vi "InitADCard.vi"(0 "task in":refnum<k21>, 1 "AD-Channels":string[](array[string]), 2 "reconfig (true)":bool=TRUE, 3 "Timing":T1={"AD-clock"=4000000.0, "external ADclock"=TRUE, "Galvocycle"=1e-05, "Bitsize"=1e-07, "AD.start.delay"=0.0, "AddStartTriggerIn"=FALSE, "VoltageRange"={"min Voltage"=-0.1, "max Voltage"=10.0}}, 4 "buffer size >1E6 (2.5E6)":i32=4000000, 5 "error in (no error)":errorcluster) -> (6 "task out":refnum<k21>, 7 "bit shifts up to 16bit":u8, 8 "error out":errorcluster)   [LabVIEW 2011]
uses:
  <vilib>/DAQmx/create/channels.llb/DAQmx Create Channel (AI-Voltage-Basic).vi
  <vilib>/DAQmx/configure/timing.llb/DAQmx Timing (Sample Clock).vi
  <vilib>/DAQmx/configure/trigger.llb/DAQmx Start Trigger (Digital Edge).vi
  National Instruments/LabVIEW 2011/resource/objmgr/daqmx.rc
panel:
  out "Trigger Pin":string
  out "8MHz Pin":string
  out "AI.RawSampJustification":i32(ring)=10279 items=["Right-Justified"=10279, "Left-Justified"=10209]
  out "RawDataWidth":u32
  out "NaN/Path/Refnum?":bool
  in  "trigger type (digital start)":enum16{"no trigger", "digital start"}(ring)=enum."digital start"
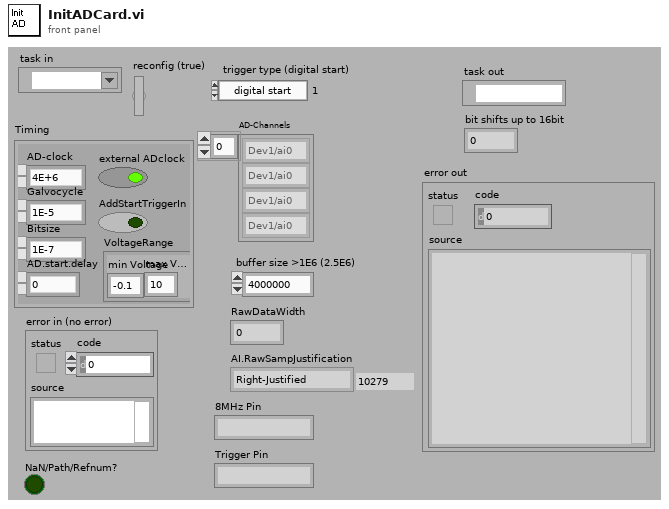
[diagram p1: front panel]
types:
  T1 = cluster{"AD-clock":dbl, "external ADclock":bool, "Galvocycle":dbl, "Bitsize":dbl, "AD.start.delay":dbl, "AddStartTriggerIn":bool, "VoltageRange":cluster{"min Voltage":dbl, "max Voltage":dbl}}
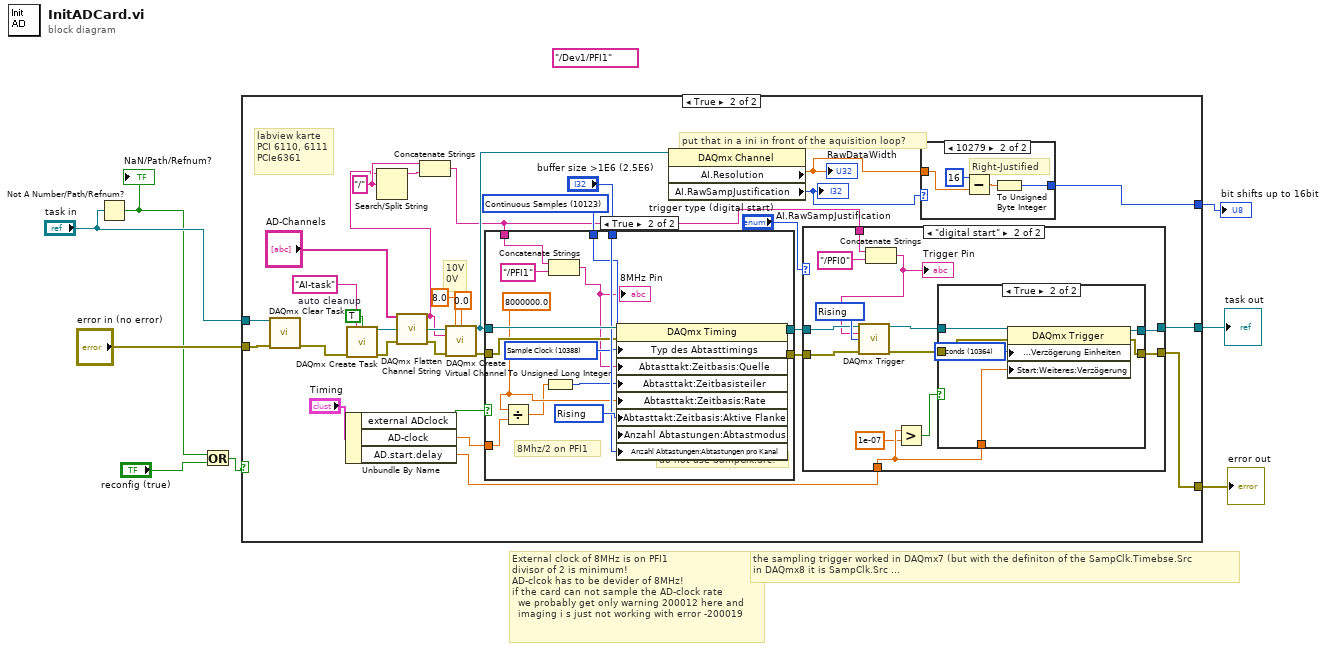
[diagram p0: block diagram]
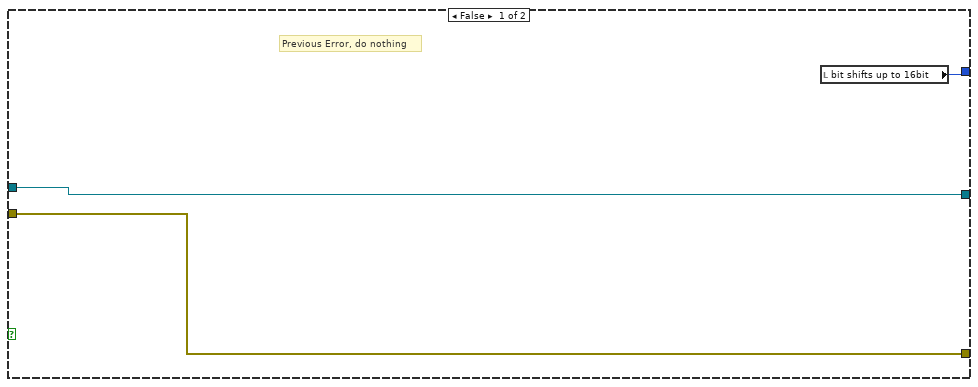
[diagram p2: hidden frame]
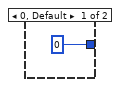
[diagram p3: hidden frame]
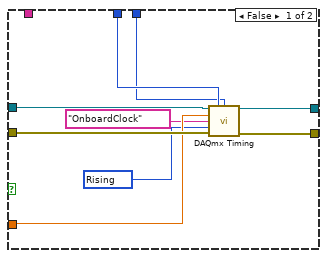
[diagram p6: hidden frame]
diagram:
  (unwired) tag "/Dev1/PFI1" ("source")
  # "External clock of 8MHz is on PFI1\ndivisor of 2 is minimum!\nAD-clcok has to be devider of 8MHz!\nif the card can not sample the AD-clock rate\n  we probably get only warning 200012 here and\n  imaging i s just not working with error -200019"
  # "the sampling trigger worked in DAQmx7 (but with the definiton of the SampClk.Timebse.Src\nin DAQmx8 it is SampClk.Src ..."
  n1 = Not A Number/Path/Refnum?(number/path/refnum="task in") -> (NaN/Path/Refnum?=w5:bool)
  "NaN/Path/Refnum?" <- w5
  n2 = Or(x=w5, y="reconfig (true)") -> (x .or. y?=w3:bool)
  n3 = case shown="True" w3 {
    tunnel: [w11 w29] -> w8
    tunnel: "error in (no error)" -> [w11 w21]
    tunnel: "task in" -> [w10 w20]
    tunnel: [w10 w23] -> w2
    tunnel: [w9 w16] -> w1
    frame False {
      # "Previous Error, do nothing"
      n4 = local read "bit shifts up to 16bit"() -> (w9:u8)
    }
    frame True {
      w14 = "/" ("search string/char (-)")
      w33 = 10123 items=["Finite Samples"=10178, "Continuous Samples"=10123, "Hardware Timed Single Point"=12522] ("sample mode")
      w41 = TRUE  # auto cleanup
      # "labview karte\nPCI 6110, 6111\nPCIe6361"
      # "put that in a ini in front of the aquisition loop?"
      # "10V\n0V"
      n5 = call <vilib>:"DAQmx Clear Task.vi"("task in"=w20, "error in"=w21) -> ("error out"=w22:errorcluster)  [unwired: 13 out]
      n6 = Unbundle By Name("Timing") -> ("external ADclock"=w26:bool, "AD-clock"=w25:dbl, "AD.start.delay"=w24:dbl)
      n7 = call <vilib>:"DAQmx Create Task.vi"("new task name"="AI-task", "auto cleanup"=w41, "error in"=w22) -> ("task out"=w40:refnum<k21>, "error out"=w38:errorcluster)  [unwired: 2 in, 9 out]
      n8 = call <vilib>:"DAQmx Flatten Channel String.vi"("names in"="AD-Channels", "error in"=w38) -> ("names out"=w13:string, "error out"=w37:errorcluster)  [unwired: 12 out]
      n9 = Search/Split String(string=w13, search string/char (-)=w14) -> (substring before match=w15:string)  [unwired: 3 out]
      n10 = Concatenate Strings(w14, w15) -> (w12:string)
      n11 = call-poly <vilib>:"DAQmx Create Virtual Channel.vi"("task in"=w40, "maximum value"=8.0, "minimum value"=0.0, "physical channels"=w13, "error in"=w37) -> ("task out"=w19:refnum<k21>, "error out"=w34:errorcluster)  [unwired: 4 in, 5 out]
      n12 = case shown="True" w26 {
        tunnel: w25 -> [w77 w85]
        tunnel: w34 -> [w78 w89]
        tunnel: w19 -> [w79 w93]
        tunnel: w33 -> [w74 w90]
        tunnel: "buffer size >1E6 (2.5E6)" -> [w73 w91]
        tunnel: [w72 w94] -> w31
        tunnel: [w71 w88] -> w30
        tunnel: w12 -> [_ w82]
        frame False {
          w76 = 10280 items=["Rising"=10280, "Falling"=10171] ("active edge")
          n13 = call-poly <vilib>:"DAQmx Timing.vi"("task/channels in"=w79, "sample mode"=w74, "samples per channel"=w73, "rate"=w77, "source"=tag "OnboardClock", "active edge"=w76, "error in"=w78) -> ("task out"=w72:refnum<k21>, "error out"=w71:errorcluster)  [unwired: 7 out]
        }
        frame True {
          w86 = 8000000.0 ("rate")
          w87 = 10388 items=["Sample Clock"=10388, "Burst Handshake"=12548, "Handshake"=10389, "Implicit"=10451, "On Demand"=10390, "Change Detection"=12504] ("SampTimingType")
          w92 = 10280 items=["Rising"=10280, "Falling"=10171] ("active edge")
          # "do not use SampClk.Src!"
          # "8Mhz/2 on PFI1"
          n14 = Divide(x=w86, y=w85) -> (x/y=w84:dbl)
          n15 = To Unsigned Long Integer(number=w84) -> (unsigned 32bit integer=w83:u32)
          n16 = Concatenate Strings(w82, "/PFI1" ("string")) -> (w80:string)
          "8MHz Pin" <- w80
          n17 = property class="DAQmx Timing"(reference=w93, error in=w89, "Typ des Abtasttimings"=w87, "Abtasttakt:Zeitbasis:Quelle"=w80, "Abtasttakt:Zeitbasisteiler"=w83, "Abtasttakt:Zeitbasis:Rate"=w86, "Abtasttakt:Zeitbasis:Aktive Flanke"=w92, "Anzahl Abtastungen:Abtastmodus"=w90, "Anzahl Abtastungen:Abtastungen pro Kanal"=w91) -> (reference out=w94:refnum<k21>, error out=w88:errorcluster)
        }
      }
      n18 = property class="DAQmx Channel"(reference=w19) -> ("AI.Resolution"=w17:dbl, "AI.RawSampJustification"=w18:i32)  [unwired: 1 in, 2 out]
      "RawDataWidth" <- w17
      "AI.RawSampJustification" <- w18
      n19 = case shown="\"digital start\"" "trigger type (digital start)" {
        tunnel: w31 -> [w49 w60]
        tunnel: w30 -> [w48 w62]
        tunnel: [w49 w55] -> w23
        tunnel: [w48 w54] -> w29
        tunnel: w24 -> [_ w59]
        tunnel: w12 -> [_ w51]
        frame "no trigger", Default {
          # "no trigger"
        }
        frame "digital start" {
          w61 = 10280 items=["Rising"=10280, "Falling"=10171] ("edge")
          # "digital A trigger"
          n20 = Concatenate Strings(w51, "/PFI0" ("string")) -> (w50:string)
          "Trigger Pin" <- w50
          n21 = call-poly <vilib>:"DAQmx Trigger.vi"("task/channels in"=w60, "source"=w50, "edge"=w61, "error in"=w62) -> ("task out"=w57:refnum<k21>, "error out"=w56:errorcluster)  [unwired: 10 out]
          n22 = Greater?(x=w59, y=1e-07) -> (0:w53:bool)
          n23 = case shown="True" w53 {
            tunnel: w59 -> [_ w69]
            tunnel: w57 -> [w64 w68]
            tunnel: w56 -> [w63 w67]
            tunnel: [w64 w66] -> w55
            tunnel: [w63 w65] -> w54
            frame False {
            }
            frame True {
              w70 = 10364 items=["Sample Clock Periods"=10286, "Seconds"=10364, "Ticks"=10304] ("Start.DelayUnits")
              n24 = property class="DAQmx Trigger"(reference=w68, error in=w67, "Start:Weiteres:Verzögerung Einheiten"=w70, "Start:Weiteres:Verzögerung"=w69) -> (reference out=w66:refnum<k21>, error out=w65:errorcluster)
            }
          }
        }
      }
      n25 = case shown="10279" w18 {
        tunnel: w17 -> [_ w47]
        tunnel: [u8 0 w44] -> w16
        frame 0, Default {
        }
        frame 10279 {
          # "Right-Justified"
          n26 = Subtract(x=u32 16, y=w47) -> (x-y=w45:dbl)
          n27 = To Unsigned Byte Integer(number=w45) -> (unsigned 8bit integer=w44:u8)
        }
      }
    }
  }
  "error out" <- w8
  "task out" <- w2
  "bit shifts up to 16bit" <- w1
